vi "Start Logic.vi"(8 "error in (no error)":errorcluster, 9 "Case name string":string, 10 "UI queue":refnum<queue>, 11 "Acq. queue in":refnum<queue>) -> (0 "error out":errorcluster, 3 "Acq. queue":refnum<queue>)   [LabVIEW 2013]
uses:
  Queue/Message Queue/Typedefs/Message Cluster.ctl
  Typedefs/PMT control functions.ctl
  Peripherals Control/Shutter/Typedefs/Shutter state.ctl
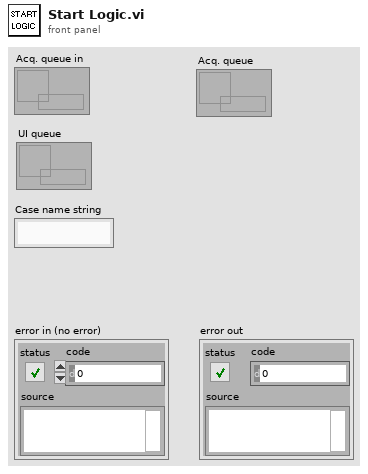
[diagram p1: front panel]
types:
  T1 = typedef "Shutter state.ctl" = enum16{"Closed/Disabled", "Open/Enabled"}
  T2 = typedef "PMT control functions.ctl" = enum16{"Set PMTs from UI", "Reset PMTs"}
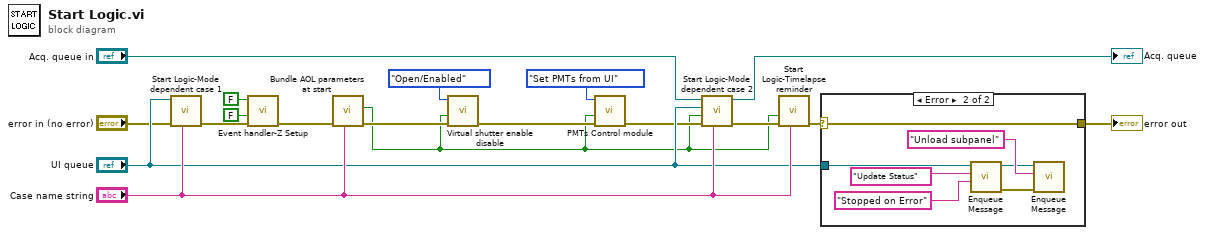
[diagram p0: block diagram]
diagram:
  n1 = call "Start Logic-Mode dependent case 1.vi"("Case name string"="Case name string", "error in (no error)"="error in (no error)", "UI queue"="UI queue") -> ("error out"=w5:errorcluster)  [unwired: 8 in]
  n2 = call "Event handler-Z Setup.vi"("error in (no error)"=w5, "Obtain Z Stop"=FALSE, "Obtain Z Start"=FALSE) -> ("error out"=w6:errorcluster)  [unwired: 8 in]
  n3 = call "Bundle AOL parameters at start.vi"("Case name string"="Case name string", "error in (no error)"=w6) -> ("error out"=w8:errorcluster, "cancelled"=w1:bool)  [unwired: 8 in]
  n4 = call "Virtual shutter enable disable.vi"("error in (no error)"=w8, "Cancelled"=w1, "Virtual Shutter"=Shutter_state."Open/Enabled") -> ("error out"=w7:errorcluster)  [unwired: 8 in]
  n5 = call "PMTs Control module.vi"("Error In"=w7, "Cancelled"=w1, "Function"=PMT_control_functions."Set PMTs from UI") -> ("Error Out"=w11:errorcluster)  [unwired: 8 in]
  n6 = call "Start Logic-Mode dependent case 2.vi"("Case name string"="Case name string", "error in (no error)"=w11, "cancelled"=w1, "UI queue"="UI queue", "Acq. queue in"="Acq. queue in") -> ("error out"=w2:errorcluster, "Acq. queue out"=→"Acq. queue":refnum<queue>)  [unwired: 5 in]
  n7 = call "Start Logic-Timelapse reminder.vi"("Case name string"="Case name string", "error in (no error)"=w2, "cancelled"=w1) -> ("error out"=w12:errorcluster)  [unwired: 8 in]
  n8 = case shown="Error" w12 {
    selector: w12 -> [_ w19]
    tunnel: "UI queue" -> [_ w20]
    tunnel: [_ w19] -> w14
    frame No Error {
    }
    frame Error {
      n9 = call "Enqueue Message.vi"("Message Data"="Stopped on Error" ("Message"), "Message"="Update Status", "Queue"=w20) -> ("error out"=w22:errorcluster, "Queue out"=w21:refnum<queue>)  [unwired: 7 in]
      n10 = call "Enqueue Message.vi"("error in (no error)"=w22, "Message"="Unload subpanel", "Queue"=w21) -> ()  [unwired: 7 in, 2 out]
    }
  }
  "error out" <- w14
